vi "Weather Parse Test.vi"() -> ()   [LabVIEW 2020, in "CDM-Config.lvlib"] (continued)
 to 60 NM\\noffshore including San Nicolas and Santa Barbara Islands.\\n\\n* WHEN...From 9 PM this evening to 2 PM PST Thursday.\\n\\n* IMPACTS...Conditions will be hazardous to small craft.\\n\\n* ADDITIONAL DETAILS...See the Coastal Waters Forecast (CWFLOX)\\nfor more.\",\n                \"instruction\": \"Inexperienced mariners, especially those operating smaller\\nvessels, should avoid navigating in hazardous conditions.\",\n                \"response\": \"Avoid\",\n                \"parameters\": {\n                    \"AWIPSidentifier\": [\n                        \"MWWLOX\"\n                    ],\n                    \"WMOidentifier\": [\n                        \"WHUS76 KLOX 031003\"\n                    ],\n                    \"NWSheadline\": [\n                        \"SMALL CRAFT ADVISORY IN EFFECT FROM 9 PM THIS EVENING TO 2 PM PST THURSDAY\"\n                    ],\n                    \"BLOCKCHANNEL\": [\n                        \"EAS\",\n                        \"NWEM\",\n                        \"CMAS\"\n                    ],\n                    \"VTEC\": [\n                        \"/O.NEW.KLOX.SC.Y.0187.251204T0500Z-251204T2200Z/\"\n                    ],\n                    \"eventEndingTime\": [\n                        \"2025-12-04T14:00:00-08:00\"\n                    ]\n                },\n                \"scope\": \"Public\",\n                \"code\": \"IPAWSv1.0\",\n                \"language\": \"en-US\",\n                \"web\": \"http://www.weather.gov\",\n                \"eventCode\": {\n                    \"SAME\": [\n                        \"NWS\"\n                    ],\n                    \"NationalWeatherService\": [\n                        \"SCY\"\n                    ]\n                }\n            }\n        },\n        {\n            \"id\": \"https://api.weather.gov/alerts/urn:oid:2.49.0.1.840.0.b223a23810f154d96d0d97456b98216ffe2bcb9d.002.1\",\n            \"type\": \"Feature\",\n            \"geometry\": null,\n            \"properties\": {\n                \"@id\": \"https://api.weather.gov/alerts/urn:oid:2.49.0.1.840.0.b223a23810f154d96d0d97456b98216ffe2bcb9d.002.1\",\n                \"@type\": \"wx:Alert\",\n                \"id\": \"urn:oid:2.49.0.1.840.0.b223a23810f154d96d0d97456b98216ffe2bcb9d.002.1\",\n                \"areaDesc\": \"Point Piedras Blancas to Point Sal from 10 to 60 NM\",\n                \"geocode\": {\n                    \"SAME\": [\n                        \"057670\"\n                    ],\n                    \"UGC\": [\n                        \"PZZ670\"\n                    ]\n                },\n                \"affectedZones\": [\n                    \"https://api.weather.gov/zones/forecast/PZZ670\"\n                ],\n                \"references\": [\n                    {\n                        \"@id\": \"https://api.weather.gov/alerts/urn:oid:2.49.0.1.840.0.da9279c8d6a996e741e643e2cbd0d5a9445846be.003.1\",\n                        \"identifier\": \"urn:oid:2.49.0.1.840.0.da9279c8d6a996e741e643e2cbd0d5a9445846be.003.1\",\n                        \"sender\": \"w-nws.webmaster@noaa.gov\",\n                        \"sent\": \"2025-12-02T21:13:00-08:00\"\n                    }\n                ],\n                \"sent\": \"2025-12-03T02:03:00-08:00\",\n                \"effective\": \"2025-12-03T02:03:00-08:00\",\n                \"onset\": \"2025-12-03T02:03:00-08:00\",\n                \"expires\": \"2025-12-03T10:00:00-08:00\",\n                \"ends\": \"2025-12-03T10:00:00-08:00\",\n                \"status\": \"Actual\",\n                \"messageType\": \"Update\",\n                \"category\": \"Met\",\n                \"severity\": \"Minor\",\n                \"certainty\": \"Likely\",\n                \"urgency\": \"Expected\",\n                \"event\": \"Small Craft Advisory\",\n                \"sender\": \"w-nws.webmaster@noaa.gov\",\n                \"senderName\": \"NWS Los Angeles/Oxnard CA\",\n                \"headline\": \"Small Craft Advisory issued December 3 at 2:03AM PST until December 3 at 10:00AM PST by NWS Los Angeles/Oxnard CA\",\n                \"description\": \"* WHAT...Hazardous sea conditions.\\n\\n* WHERE...Point Piedras Blancas to Point Sal from 10 to 60 NM.\\n\\n* WHEN...Until 10 AM PST this morning.\\n\\n* IMPACTS...Conditions will be hazardous to small craft.\\n\\n* ADDITIONAL DETAILS...See the Coastal Waters Forecast (CWFLOX)\\nfor more.\",\n                \"instruction\": \"Inexperienced mariners, especially those operating smaller\\nvessels, should avoid navigating in hazardous conditions.\",\n                \"response\": \"Avoid\",\n                \"parameters\": {\n                    \"AWIPSidentifier\": [\n                        \"MWWLOX\"\n                    ],\n                    \"WMOidentifier\": [\n                        \"WHUS76 KLOX 031003\"\n                    ],\n                    \"NWSheadline\": [\n                        \"SMALL CRAFT ADVISORY REMAINS IN EFFECT UNTIL 10 AM PST THIS MORNING\"\n                    ],\n                    \"BLOCKCHANNEL\": [\n                        \"EAS\",\n                        \"NWEM\",\n                        \"CMAS\"\n                    ],\n                    \"VTEC\": [\n                        \"/O.CON.KLOX.SC.Y.0186.000000T0000Z-251203T1800Z/\"\n                    ],\n                    \"eventEndingTime\": [\n                        \"2025-12-03T10:00:00-08:00\"\n                    ],\n                    \"expiredReferences\": [\n                        \"w-nws.webmaster@noaa.gov,urn:oid:2.49.0.1.840.0.03bf4d8e76a679c68e6d6d1c69bed8b6ac358ac0.001.1,2025-12-02T16:31:00-08:00 w-nws.webmaster@noaa.gov,urn:oid:2.49.0.1.840.0.a0fbc3255ee7827afecade81522465af6da1e5e8.001.1,2025-12-02T08:16:00-08:00 w-nws.webmaster@noaa.gov,urn:oid:2.49.0.1.840.0.8e668e000c4ef90085bd20b8852b2e419ef5ec00.001.1,2025-12-02T02:02:00-08:00\"\n                    ]\n                },\n                \"scope\": \"Public\",\n                \"code\": \"IPAWSv1.0\",\n                \"language\": \"en-US\",\n                \"web\": \"http://www.weather.gov\",\n                \"eventCode\": {\n                    \"SAME\": [\n                        \"NWS\"\n                    ],\n                    \"NationalWeatherService\": [\n                        \"SCY\"\n                    ]\n                }\n            }\n        },\n        {\n            \"id\": \"https://api.weather.gov/alerts/urn:oid:2.49.0.1.840.0.71d851f215deadf32c950ba049a11b63260bba93.001.1\",\n            \"type\": \"Feature\",\n            \"geometry\": null,\n            \"properties\": {\n                \"@id\": \"https://api.weather.gov/alerts/urn:oid:2.49.0.1.840.0.71d851f215deadf32c950ba049a11b63260bba93.001.1\",\n                \"@type\": \"wx:Alert\",\n                \"id\": \"urn:oid:2.49.0.1.840.0.71d851f215deadf32c950ba049a11b63260bba93.001.1\",\n                \"areaDesc\": \"Columbia River Bar\",\n                \"geocode\": {\n                    \"SAME\": [\n                        \"057210\"\n                    ],\n                    \"UGC\": [\n                        \"PZZ210\"\n                    ]\n                },\n                \"affectedZones\": [\n                    \"https://api.weather.gov/zones/forecast/PZZ210\"\n                ],\n                \"references\": [],\n                \"sent\": \"2025-12-03T02:01:00-08:00\",\n                \"effective\": \"2025-12-03T02:01:00-08:00\",\n                \"onset\": \"2025-12-03T13:00:00-08:00\",\n                \"expires\": \"2025-12-03T17:00:00-08:00\",\n                \"ends\": \"2025-12-03T17:00:00-08:00\",\n                \"status\": \"Actual\",\n                \"messageType\": \"Alert\",\n                \"category\": \"Met\",\n                \"severity\": \"Minor\",\n                \"certainty\": \"Likely\",\n                \"urgency\": \"Expected\",\n                \"event\": \"Small Craft Advisory\",\n                \"sender\": \"w-nws.webmaster@noaa.gov\",\n                \"senderName\": \"NWS Portland OR\",\n                \"headline\": \"Small Craft Advisory issued December 3 at 2:01AM PST until December 3 at 5:00PM PST by NWS Portland OR\",\n                \"description\": \"* WHAT...Rough bar conditions expected during a very strong ebb\\ncurrent of 7.14 kt at 301 PM Wednesday. Seas 10 ft.\\n\\n* WHERE...In the Main Channel of the Columbia River Bar.\\n\\n* WHEN...From 1 PM to 5 PM PST this afternoon.\\n\\n* IMPACTS...Conditions will be hazardous to small craft,\\nespecially when operating near to, or attempting to cross, the\\nColumbia River Bar.\",\n                \"instruction\": \"A Small Craft Advisory means that wave conditions are expected to\\nbe hazardous to small craft in the vicinity of the Columbia River\\nBar. Mariners are advised to obtain the latest bar conditions\\nfrom the United States Coast Guard before attempting to cross the\\nbar.\",\n                \"response\": \"Avoid\",\n                \"parameters\": {\n                    \"AWIPSidentifier\": [\n                        \"MWWPQR\"\n                    ],\n                    \"WMOidentifier\": [\n                        \"WHUS76 KPQR 031001\"\n                    ],\n                    \"NWSheadline\": [\n                        \"SMALL CRAFT ADVISORY IN EFFECT FROM 1 PM TO 5 PM PST THIS AFTERNOON\"\n                    ],\n                    \"BLOCKCHANNEL\": [\n                        \"EAS\",\n                        \"NWEM\",\n                        \"CMAS\"\n                    ],\n                    \"VTEC\": [\n                        \"/O.NEW.KPQR.SC.Y.0142.251203T2100Z-251204T0100Z/\"\n                    ],\n                    \"eventEndingTime\": [\n                        \"2025-12-03T17:00:00-08:00\"\n                    ]\n                },\n                \"scope\": \"Public\",\n                \"code\": \"IPAWSv1.0\",\n                \"language\": \"en-US\",\n                \"web\": \"http://www.weather.gov\",\n                \"eventCode\": {\n                    \"SAME\": [\n                        \"NWS\"\n                    ],\n                    \"NationalWeatherService\": [\n                        \"SCY\"\n                    ]\n                }\n            }\n        },\n        {\n            \"id\": \"https://api.weather.gov/alerts/urn:oid:2.49.0.1.840.0.b40606fb01e4d94a8ca9e9a27f2c4722d3eb8aec.002.1\",\n            \"type\": \"Feature\",\n            \"geometry\": null,\n            \"properties\": {\n                \"@id\": \"https://api.weather.gov/alerts/urn:oid:2.49.0.1.840.0.b40606fb01e4d94a8ca9e9a27f2c4722d3eb8aec.002.1\",\n                \"@type\": \"wx:Alert\",\n                \"id\": \"urn:oid:2.49.0.1.840.0.b40606fb01e4d94a8ca9e9a27f2c4722d3eb8aec.002.1\",\n                \"areaDesc\": \"Tillamook County Coast; Central Coast of Oregon\",\n                \"geocode\": {\n                    \"SAME\": [\n                        \"041057\",\n                        \"041041\",\n                        \"041039\"\n                    ],\n                    \"UGC\": [\n                        \"ORZ102\",\n                        \"ORZ103\"\n                    ]\n                },\n                \"affectedZones\": [\n                    \"https://api.weather.gov/zones/forecast/ORZ102\",\n                    \"https://api.weather.gov/zones/forecast/ORZ103\"\n                ],\n                \"references\": [\n                    {\n                        \"@id\": \"https://api.weather.gov/alerts/urn:oid:2.49.0.1.840.0.b0d8924765acde472ad27290e55ee6e4f32b14ec.002.1\",\n                        \"identifier\": \"urn:oid:2.49.0.1.840.0.b0d8924765acde472ad27290e55ee6e4f32b14ec.002.1\",\n                        \"sender\": \"w-nws.webmaster@noaa.gov\",\n                        \"sent\": \"2025-12-02T15:12:00-08:00\"\n                    }\n                ],\n                \"sent\": \"2025-12-03T02:01:00-08:00\",\n                \"effective\": \"2025-12-03T02:01:00-08:00\",\n                \"onset\": \"2025-12-03T02:01:00-08:00\",\n                \"expires\": \"2025-12-03T22:00:00-08:00\",\n                \"ends\": \"2025-12-03T22:00:00-08:00\",\n                \"status\": \"Actual\",\n                \"messageType\": \"Update\",\n                \"category\": \"Met\",\n                \"severity\": \"Moderate\",\n                \"certainty\": \"Likely\",\n                \"urgency\": \"Expected\",\n                \"event\": \"Beach Hazards Statement\",\n                \"sender\": \"w-nws.webmaster@noaa.gov\",\n                \"senderName\": \"NWS Portland OR\",\n                \"headline\": \"Beach Hazards Statement issued December 3 at 2:01AM PST until December 3 at 10:00PM PST by NWS Portland OR\",\n                \"description\": \"* WHAT...Sneaker waves possible.\\n\\n* WHERE...Tillamook County Coast and Central Coast of Oregon.\\n\\n* WHEN...Through this evening.\\n\\n* IMPACTS...Waves can run up significantly farther on a beach\\nthan normal, including over rocks and jetties. Sneaker waves\\ncan suddenly knock beachgoers off if their feet and quickly\\npull them into the frigid ocean which may lead to serious\\ninjury or drowning.\\n\\n* ADDITIONAL DETAILS...A Beach Hazards Statement is issued when\\nsneaker waves create potentially life-threatening conditions\\nin the surf zone. Caution should be used when in or near the\\nwater. Always keep an eye on the waves, and be especially\\nwatchful of children. Those participating in razor clam digs\\nshould additionally exercise caution.\",\n                \"instruction\": \"Remain out of the water to avoid hazardous swimming conditions.\",\n                \"response\": \"Avoid\",\n                \"parameters\": {\n                    \"AWIPSidentifier\": [\n                        \"CFWPQR\"\n                    ],\n                    \"WMOidentifier\": [\n                        \"WHUS46 KPQR 031001\"\n                    ],\n                    \"NWSheadline\": [\n                        \"BEACH HAZARDS STATEMENT REMAINS IN EFFECT THROUGH THIS EVENING\"\n                    ],\n                    \"BLOCKCHANNEL\": [\n                        \"EAS\",\n                        \"NWEM\",\n                        \"CMAS\"\n                    ],\n                    \"VTEC\": [\n                        \"/O.CON.KPQR.BH.S.0016.000000T0000Z-251204T0600Z/\"\n                    ],\n                    \"eventEndingTime\": [\n                        \"2025-12-03T22:00:00-08:00\"\n                    ],\n                    \"expiredReferences\": [\n                        \"w-nws.webmaster@noaa.gov,urn:oid:2.49.0.1.840.0.4a86d466bdedede9df987ed309d495de11850650.001.1,2025-12-01T14:28:00-08:00 w-nws.webmaster@noaa.gov,urn:oid:2.49.0.1.840.0.7f5d42e9aa955b7ce231997bb6cbc5205d11387b.001.1,2025-11-30T13:55:00-08:00 w-nws.webmaster@noaa.gov,urn:oid:2.49.0.1.840.0.f9f5603af29c238f0de04ac7e2a9349708c05a53.001.1,2025-11-29T13:40:00-08:00 w-nws.webmaster@noaa.gov,urn:oid:2.49.0.1.840.0.5d50b6fb5ef96869ff9b56cca9e1ba6ccd50c4dd.001.1,2025-11-28T14:00:00-08:00\"\n                    ]\n                },\n                \"scope\": \"Public\",\n                \"code\": \"IPAWSv1.0\",\n                \"language\": \"en-US\",\n                \"web\": \"http://www.weather.gov\",\n                \"eventCode\": {\n                    \"SAME\": [\n                        \"NWS\"\n                    ],\n                    \"NationalWeatherService\": [\n                        \"BHS\"\n                    ]\n                }\n            }\n        },\n        {\n            \"id\": \"https://api.weather.gov/alerts/urn:oid:2.49.0.1.840.0.b40606fb01e4d94a8ca9e9a27f2c4722d3eb8aec.001.1\",\n            \"type\": \"Feature\",\n            \"geometry\": null,\n            \"properties\": {\n                \"@id\": \"https://api.weather.gov/alerts/urn:oid:2.49.0.1.840.0.b40606fb01e4d94a8ca9e9a27f2c4722d3eb8aec.001.1\",\n                \"@type\": \"wx:Alert\",\n                \"id\": \"urn:oid:2.49.0.1.840.0.b40606fb01e4d94a8ca9e9a27f2c4722d3eb8aec.001.1\",\n                \"areaDesc\": \"Clatsop County Coast; South Washington Coast\",\n                \"geocode\": {\n                    \"SAME\": [\n                        \"041007\",\n                        \"053049\"\n                    ],\n                    \"UGC\": [\n                        \"ORZ101\",\n                        \"WAZ201\"\n                    ]\n                },\n                \"affectedZones\": [\n                    \"https://api.weather.gov/zones/forecast/ORZ101\",\n                    \"https://api.weather.gov/zones/forecast/WAZ201\"\n                ],\n                \"references\": [\n                    {\n                        \"@id\": \"https://api.weather.gov/alerts/urn:oid:2.49.0.1.840.0.b0d8924765acde472ad27290e55ee6e4f32b14ec.001.1\",\n                        \"identifier\": \"urn:oid:2.49.0.1.840.0.b0d8924765acde472ad27290e55ee6e4f32b14ec.001.1\",\n                        \"sender\": \"w-nws.webmaster@noaa.gov\",\n                        \"sent\": \"2025-12-02T15:12:00-08:00\"\n                    }\n                ],\n                \"sent\": \"2025-12-03T02:01:00-08:00\",\n                \"effective\": \"2025-12-03T02:01:00-08:00\",\n                \"onset\": \"2025-12-04T09:00:00-08:00\",\n                \"expires\": \"2025-12-03T22:00:00-08:00\",\n                \"ends\": \"2025-12-04T14:00:00-08:00\",\n                \"status\": \"Actual\",\n                \"messageType\": \"Update\",\n                \"category\": \"Met\",\n                \"severity\": \"Minor\",\n                \"certainty\": \"Likely\",\n                \"urgency\": \"Expected\",\n                \"event\": \"Coastal Flood Advisory\",\n                \"sender\": \"w-nws.webmaster@noaa.gov\",\n                \"senderName\": \"NWS Portland OR\",\n                \"headline\": \"Coastal Flood Advisory issued December 3 at 2:01AM PST until December 4 at 2:00PM PST by NWS Portland OR\",\n                \"description\": \"* WHAT...For the Beach Hazards Statement, Sneaker waves\\npossible. For the Coastal Flood Advisory, tidal overflow\\nflooding expected.\\n\\n* WHERE...In Oregon, Clatsop County Coast. In Washington, South\\nWashington Coast.\\n\\n* WHEN...For the Beach Hazards Statement, through this evening.\\nFor the Coastal Flood Advisory, from 9 AM to 2 PM PST Thursday.\\n\\n* IMPACTS...Waves can run up significantly farther on a beach\\nthan normal, including over rocks and jetties. Sneaker waves\\ncan suddenly knock beachgoers off if their feet and quickly\\npull them into the frigid ocean which may lead to serious\\ninjury or drowning.\\n\\nFor the Coastal Flood Advisory, minor flooding is possible in\\nlow lying areas near bays, sloughs, and the lower reaches of\\nthe coastal rivers. This is due to total tide of up to 11.1\\nfeet at Toke Point resulting in tide up to one foot above\\nground level during high tide, total tide of up to 10.6 feet\\nat Tongue Point resulting in tide up to one foot above ground\\nlevel.\\n\\n* ADDITIONAL DETAILS...A Beach Hazards Statement is issued when\\nsneaker waves create potentially life-threatening conditions\\nin the surf zone. Caution should be used when in or near the\\nwater. Always keep an eye on the waves, and be especially\\nwatchful of children. Those participating in razor clam digs\\nshould additionally exercise caution.\",\n                \"instruction\": \"A Coastal Flood Advisory means that tidal overflow flooding is\\nexpected. Coastal residents in the warned area should be alert\\nfor rising water, and take appropriate action to protect life and\\nproperty.\\n\\nRemain out of the water to avoid hazardous swimming conditions.\",\n                \"response\": \"Monitor\",\n                \"parameters\": {\n                    \"AWIPSidentifier\": [\n                        \"CFWPQR\"\n                    ],\n                    \"WMOidentifier\": [\n                        \"WHUS46 KPQR 031001\"\n                    ],\n                    \"NWSheadline\": [\n                        \"BEACH HAZARDS STATEMENT REMAINS IN EFFECT THROUGH THIS EVENING... ...COASTAL FLOOD ADVISORY REMAINS IN EFFECT FROM 9 AM TO 2 PM PST THURSDAY\"\n                    ],\n                    \"BLOCKCHANNEL\": [\n                        \"EAS\",\n                        \"NWEM\",\n                        \"CMAS\"\n                    ],\n                    \"VTEC\": [\n                        \"/O.CON.KPQR.CF.Y.0005.251204T1700Z-251204T2200Z/\"\n                    ],\n                    \"eventEndingTime\": [\n                        \"2025-12-04T14:00:00-08:00\"\n                    ]\n                },\n                \"scope\": \"Public\",\n                \"code\": \"IPAWSv1.0\",\n                \"language\": \"en-US\",\n                \"web\": \"http://www.weather.gov\",\n                \"eventCode\": {\n                    \"SAME\": [\n                        \"NWS\"\n                    ],\n                    \"NationalWeatherService\": [\n                        \"CFY\"\n                    ]\n                }\n            }\n        },\n        {\n            \"id\": \"https://api.weather.gov/alerts/urn:oid:2.49.0.1.840.0.b40606fb01e4d94a8ca9e9a27f2c4722d3eb8aec.001.2\",\n            \"type\": \"Feature\",\n            \"geometry\": null,\n            \"properties\": {\n                \"@id\": \"https://api.weather.gov/alerts/urn:oid:2.49.0.1.840.0.b40606fb01e4d94a8ca9e9a27f2c4722d3eb8aec.001.2\",\n                \"@type\": \"wx:Alert\",\n                \"id\": \"urn:oid:2.49.0.1.840.0.b40606fb01e4d94a8ca9e9a27f2c4722d3eb8aec.001.2\",\n                \"areaDesc\": \"Clatsop County Coast; South Washington Coast\",\n                \"geocode\": {\n                    \"SAME\": [\n                        \"041007\",\n                        \"053049\"\n                    ],\n                    \"UGC\": [\n                        \"ORZ101\",\n                        \"WAZ201\"\n                    ]\n                },\n                \"affectedZones\": [\n                    \"https://api.weather.gov/zones/forecast/ORZ101\",\n                    \"https://api.weather.gov/zones/forecast/WAZ201\"\n                ],\n                \"references\": [\n                    {\n                        \"@id\": \"https://api.weather.gov/alerts/urn:oid:2.49.0.1.840.0.b0d8924765acde472ad27290e55ee6e4f32b14ec.001.2\",\n                        \"identifier\": \"urn:oid:2.49.0.1.840.0.b0d8924765acde472ad27290e55ee6e4f32b14ec.001.2\",\n                        \"sender\": \"w-nws.webmaster@noaa.gov\",\n                        \"sent\": \"2025-12-02T15:12:00-08:00\"\n                    }\n                ],\n                \"sent\": \"2025-12-03T02:01:00-08:00\",\n                \"effective\": \"2025-12-03T02:01:00-08:00\",\n                \"onset\": \"2025-12-03T02:01:00-08:00\",\n                \"expires\": \"2025-12-03T22:00:00-08:00\",\n                \"ends\": \"2025-12-03T22:00:00-08:00\",\n                \"status\": \"Actual\",\n                \"messageType\": \"Update\",\n                \"category\": \"Met\",\n                \"severity\": \"Moderate\",\n                \"certainty\": \"Likely\",\n                \"urgency\": \"Expected\",\n                \"event\": \"Beach Hazards Statement\",\n                \"sender\": \"w-nws.webmaster@noaa.gov\",\n                \"senderName\": \"NWS Portland OR\",\n                \"headline\": \"Beach Hazards Statement issued December 3 at 2:01AM PST until December 3 at 10:00PM PST by NWS Portland OR\",\n                \"description\": \"* WHAT...For the Beach Hazards Statement, Sneaker waves\\npossible. For the Coastal Flood Advisory, tidal overflow\\nflooding expected.\\n\\n* WHERE...In Oregon, Clatsop County Coast. In Washington, South\\nWashington Coast.\\n\\n* WHEN...For the Beach Hazards Statement, through this evening.\\nFor the Coastal Flood Advisory, from 9 AM to 2 PM PST Thursday.\\n\\n* IMPACTS...Waves can run up significantly farther on a beach\\nthan normal, including over rocks and jetties. Sneaker waves\\ncan suddenly knock beachgoers off if their feet and quickly\\npull them into the frigid ocean which may lead to serious\\ninjury or drowning.\\n\\nFor the Coastal Flood Advisory, minor flooding is possible in\\nlow lying areas near bays, sloughs, and the lower reaches of\\nthe coastal rivers. This is due to total tide of up to 11.1\\nfeet at Toke Point resulting in tide up to one foot above\\nground level during high tide, total tide of up to 10.6 feet\\nat Tongue Point resulting in tide up to one foot above ground\\nlevel.\\n\\n* ADDITIONAL DETAILS...A Beach Hazards Statement is issued when\\nsneaker waves create potentially life-threatening conditions\\nin the surf zone. Caution should be used when in or near the\\nwater. Always keep an eye on the waves, and be especially\\nwatchful of children. Those participating in razor clam digs\\nshould additionally exercise caution.\",\n                \"instruction\": \"A Coastal Flood Advisory means that tidal overflow flooding is\\nexpected. Coastal residents in the warned area should be alert\\nfor rising water, and take appropriate action to protect life and\\nproperty.\\n\\nRemain out of the water to avoid hazardous swimming conditions.\",\n                \"response\": \"Avoid\",\n                \"parameters\": {\n                    \"AWIPSidentifier\": [\n                        \"CFWPQR\"\n                    ],\n                    \"WMOidentifier\": [\n                        \"WHUS46 KPQR 031001\"\n                    ],\n                    \"NWSheadline\": [\n                        \"BEACH HAZARDS STATEMENT REMAINS IN EFFECT THROUGH THIS EVENING... ...COASTAL FLOOD ADVISORY REMAINS IN EFFECT FROM 9 AM TO 2 PM PST THURSDAY\"\n                    ],\n                    \"BLOCKCHANNEL\": [\n                        \"EAS\",\n                        \"NWEM\",\n                        \"CMAS\"\n                    ],\n                    \"VTEC\": [\n                        \"/O.CON.KPQR.BH.S.0016.000000T0000Z-251204T0600Z/\"\n                    ],\n                    \"eventEndingTime\": [\n                        \"2025-12-03T22:00:00-08:00\"\n                    ],\n                    \"expiredReferences\": [\n                        \"w-nws.webmaster@noaa.gov,urn:oid:2.49.0.1.840.0.4a86d466bdedede9df987ed309d495de11850650.001.1,2025-12-01T14:28:00-08:00 w-nws.webmaster@noaa.gov,urn:oid:2.49.0.1.840.0.7f5d42e9aa955b7ce231997bb6cbc5205d11387b.001.1,2025-11-30T13:55:00-08:00 w-nws.webmaster@noaa.gov,urn:oid:2.49.0.1.840.0.f9f5603af29c238f0de04ac7e2a9349708c05a53.001.1,2025-11-29T13:40:00-08:00 w-nws.webmaster@noaa.gov,urn:oid:2.49.0.1.840.0.5d50b6fb5ef96869ff9b56cca9e1ba6ccd50c4dd.001.1,2025-11-28T14:00:00-08:00\"\n                    ]\n                },\n                \"scope\": \"Public\",\n                \"code\": \"IPAWSv1.0\",\n                \"language\": \"en-US\",\n                \"web\": \"http://www.weather.gov\",\n                \"eventCode\": {\n                    \"SAME\": [\n                        \"NWS\"\n                    ],\n                    \"NationalWeatherService\": [\n                        \"BHS\"\n                    ]\n                }\n            }\n        },\n        {\n            \"id\": \"https://api.weather.gov/alerts/urn:oid:2.49.0.1.840.0.59f39e0a7f6acf285dcd268db360e347a0a8a808.001.2\",\n            \"type\": \"Feature\",\n            \"geometry\": null,\n            \"properties\": {\n                \"@id\": \"https://api.weather.gov/alerts/urn:oid:2.49.0.1.840.0.59f39e0a7f6acf285dcd268db360e347a0a8a808.001.2\",\n                \"@type\": \"wx:Alert\",\n                \"id\": \"urn:oid:2.49.0.1.840.0.59f39e0a7f6acf285dcd268db360e347a0a8a808.001.2\",\n                \"areaDesc\": \"Ventura County Beaches\",\n                \"geocode\": {\n                    \"SAME\": [\n                        \"006111\"\n                    ],\n                    \"UGC\": [\n                        \"CAZ354\"\n                    ]\n                },\n                \"affectedZones\": [\n                    \"https://api.weather.gov/zones/forecast/CAZ354\"\n                ],\n                \"references\": [\n                    {\n                        \"@id\": \"https://api.weather.gov/alerts/urn:oid:2.49.0.1.840.0.93417926f6a4e3b4090235b97e1fee71b07b4e44.001.2\",\n                        \"identifier\": \"urn:oid:2.49.0.1.840.0.93417926f6a4e3b4090235b97e1fee71b07b4e44.001.2\",\n                        \"sender\": \"w-nws.webmaster@noaa.gov\",\n                        \"sent\": \"2025-12-02T13:27:00-08:00\"\n                    }\n                ],\n                \"sent\": \"2025-12-03T02:00:00-08:00\",\n                \"effective\": \"2025-12-03T02:00:00-08:00\",\n                \"onset\": \"2025-12-03T03:00:00-08:00\",\n                \"expires\": \"2025-12-03T10:00:00-08:00\",\n                \"ends\": \"2025-12-03T10:00:00-08:00\",\n                \"status\": \"Actual\",\n                \"messageType\": \"Update\",\n                \"category\": \"Met\",\n                \"severity\": \"Minor\",\n                \"certainty\": \"Likely\",\n                \"urgency\": \"Expected\",\n                \"event\": \"Coastal Flood Advisory\",\n                \"sender\": \"w-nws.webmaster@noaa.gov\",\n                \"senderName\": \"NWS Los Angeles/Oxnard CA\",\n                \"headline\": \"Coastal Flood Advisory issued December 3 at 2:00AM PST until December 3 at 10:00AM PST by NWS Los Angeles/Oxnard CA\",\n                \"description\": \"* WHAT...For the High Surf Advisory, large breaking waves of 4 to\\n7 feet. Dangerous rip currents expected. For the Coastal Flood\\nAdvisory, minor coastal flooding is possible during high tide.\\n\\n* WHERE...Ventura County Beaches.\\n\\n* WHEN...For the High Surf Advisory, until noon PST Thursday.\\nFor the Coastal Flood Advisory, until 10 AM PST this morning.\\n\\n* IMPACTS...Flooding of sea water is likely, around the time of\\nhigh tide, over vulnerable low-lying coastal areas such as\\nparking lots, beaches, and walkways. Significant damage to roads\\nor structures is NOT expected. There is an increased risk for\\nocean drowning. Rip currents can pull swimmers and surfers out\\nto sea. Large breaking waves can cause injury, wash people off\\nbeaches and rocks, and capsize small boats near shore.\",\n                \"instruction\": \"Take the necessary actions to protect flood-prone property. Do\\nNOT drive around barricades or through water of unknown depth.\\n\\nRemain out of the water due to dangerous surf conditions, or stay\\nnear occupied lifeguard towers. Rock jetties can be deadly in\\nsuch conditions, stay off the rocks.\",\n                \"response\": \"Monitor\",\n                \"parameters\": {\n                    \"AWIPSidentifier\": [\n                        \"CFWLOX\"\n                    ],\n                    \"WMOidentifier\": [\n                        \"WHUS46 KLOX 031000\"\n                    ],\n                    \"NWSheadline\": [\n                        \"HIGH SURF ADVISORY REMAINS IN EFFECT UNTIL NOON PST THURSDAY... ...COASTAL FLOOD ADVISORY REMAINS IN EFFECT UNTIL 10 AM PST THIS MORNING\"\n                    ],\n                    \"BLOCKCHANNEL\": [\n                        \"EAS\",\n                        \"NWEM\",\n                        \"CMAS\"\n                    ],\n                    \"VTEC\": [\n                        \"/O.CON.KLOX.CF.Y.0004.251203T1100Z-251203T1800Z/\"\n                    ],\n                    \"eventEndingTime\": [\n                        \"2025-12-03T10:00:00-08:00\"\n                    ],\n                    \"expiredReferences\": [\n                        \"w-nws.webmaster@noaa.gov,urn:oid:2.49.0.1.840.0.2ef03bba301f3aa5d410947a3c0b158da4ab8a14.001.2,2025-12-02T01:44:00-08:00 w-nws.webmaster@noaa.gov,urn:oid:2.49.0.1.840.0.ca1df4acb1d2f6b371b32e7cbfbf7966eb5b8a28.001.2,2025-12-01T19:11:00-08:00 w-nws.webmaster@noaa.gov,urn:oid:2.49.0.1.840.0.9f5f82a93112b0fbb919461d7f3c09a028cde467.001.1,2025-12-01T12:55:00-08:00\"\n                    ]\n                },\n                \"scope\": \"Public\",\n                \"code\": \"IPAWSv1.0\",\n                \"language\": \"en-US\",\n                \"web\": \"http://www.weather.gov\",\n                \"eventCode\": {\n                    \"SAME\": [\n                        \"NWS\"\n                    ],\n                    \"NationalWeatherService\": [\n                        \"CFY\"\n                    ]\n                }\n            }\n        },\n        {\n            \"id\": \"https://api.weather.gov/alerts/urn:oid:2.49.0.1.840.0.59f39e0a7f6acf285dcd268db360e347a0a8a808.003.1\",\n            \"type\": \"Feature\",\n            \"geometry\": null,\n            \"properties\": {\n                \"@id\": \"https://api.weather.gov/alerts/urn:oid:2.49.0.1.840.0.59f39e0a7f6acf285dcd268db360e347a0a8a808.003.1\",\n                \"@type\": \"wx:Alert\",\n                \"id\": \"urn:oid:2.49.0.1.840.0.59f39e0a7f6acf285dcd268db360e347a0a8a808.003.1\",\n                \"areaDesc\": \"Santa Barbara County Southwestern Coast; Santa Barbara County Southeastern Coast; Malibu Coast; Los Angeles County Beaches\",\n                \"geocode\": {\n                    \"SAME\": [\n                        \"006083\",\n                        \"006037\"\n                    ],\n                    \"UGC\": [\n                        \"CAZ349\",\n                        \"CAZ350\",\n                        \"CAZ362\",\n                        \"CAZ366\"\n                    ]\n                },\n                \"affectedZones\": [\n                    \"https://api.weather.gov/zones/forecast/CAZ349\",\n                    \"https://api.weather.gov/zones/forecast/CAZ350\",\n                    \"https://api.weather.gov/zones/forecast/CAZ362\",\n                    \"https://api.weather.gov/zones/forecast/CAZ366\"\n                ],\n                \"references\": [\n                    {\n                        \"@id\": \"https://api.weather.gov/alerts/urn:oid:2.49.0.1.840.0.93417926f6a4e3b4090235b97e1fee71b07b4e44.003.1\",\n                        \"identifier\": \"urn:oid:2.49.0.1.840.0.93417926f6a4e3b4090235b97e1fee71b07b4e44.003.1\",\n                        \"sender\": \"w-nws.webmaster@noaa.gov\",\n                        \"sent\": \"2025-12-02T13:27:00-08:00\"\n                    }\n                ],\n                \"sent\": \"2025-12-03T02:00:00-08:00\",\n                \"effective\": \"2025-12-03T02:00:00-08:00\",\n                \"onset\": \"2025-12-03T02:00:00-08:00\",\n                \"expires\": \"2025-12-03T10:00:00-08:00\",\n                \"ends\": \"2025-12-06T11:00:00-08:00\",\n                \"status\": \"Actual\",\n                \"messageType\": \"Update\",\n                \"category\": \"Met\",\n                \"severity\": \"Moderate\",\n                \"certainty\": \"Likely\",\n                \"urgency\": \"Expected\",\n                \"event\": \"Beach Hazards Statement\",\n                \"sender\": \"w-nws.webmaster@noaa.gov\",\n                \"senderName\": \"NWS Los Angeles/Oxnard CA\",\n                \"headline\": \"Beach Hazards Statement issued December 3 at 2:00AM PST until December 6 at 11:00AM PST by NWS Los Angeles/Oxnard CA\",\n                \"description\": \"* WHAT...Dangerous rip currents and breaking waves due to\\nelevated surf expected. Minor tidal overflows are possible\\nfrom 4 AM to 12 PM each day through Saturday morning.\\n\\n* WHERE...Santa Barbara County Southwestern Coast, Santa Barbara\\nCounty Southeastern Coast, Malibu Coast and Los Angeles County\\nBeaches.\\n\\n* WHEN...Through Saturday morning.\\n\\n* IMPACTS...There is an increased risk of ocean drowning. Rip\\ncurrents can pull swimmers and surfers out to sea. Waves can\\nwash people off beaches and rocks, and capsize small boats\\nnearshore.\\n\\n* ADDITIONAL DETAILS... Elevated surf will be highest through\\nThursday.\",\n                \"instruction\": \"Remain out of the water due to hazardous swimming conditions, or\\nstay near occupied lifeguard towers. Rock jetties can be deadly\\nin such conditions, stay off the rocks.\",\n                \"response\": \"Avoid\",\n                \"parameters\": {\n                    \"AWIPSidentifier\": [\n                        \"CFWLOX\"\n                    ],\n                    \"WMOidentifier\": [\n                        \"WHUS46 KLOX 031000\"\n                    ],\n                    \"NWSheadline\": [\n                        \"BEACH HAZARDS STATEMENT REMAINS IN EFFECT THROUGH SATURDAY MORNING\"\n                    ],\n                    \"BLOCKCHANNEL\": [\n                        \"EAS\",\n                        \"NWEM\",\n                        \"CMAS\"\n                    ],\n                    \"VTEC\": [\n                        \"/O.CON.KLOX.BH.S.0018.000000T0000Z-251206T1900Z/\"\n                    ],\n                    \"eventEndingTime\": [\n                        \"2025-12-06T11:00:00-08:00\"\n                    ],\n                    \"expiredReferences\": [\n                        \"w-nws.webmaster@noaa.gov,urn:oid:2.49.0.1.840.0.2ef03bba301f3aa5d410947a3c0b158da4ab8a14.003.1,2025-12-02T01:44:00-08:00 w-nws.webmaster@noaa.gov,urn:oid:2.49.0.1.840.0.ca1df4acb1d2f6b371b32e7cbfbf7966eb5b8a28.003.1,2025-12-01T19:11:00-08:00 w-nws.webmaster@noaa.gov,urn:oid:2.49.0.1.840.0.9f5f82a93112b0fbb919461d7f3c09a028cde467.003.1,2025-12-01T12:55:00-08:00\"\n                    ]\n                },\n                \"scope\": \"Public\",\n                \"code\": \"IPAWSv1.0\",\n                \"language\": \"en-US\",\n                \"web\": \"http://www.weather.gov\",\n                \"eventCode\": {\n                    \"SAME\": [\n                        \"NWS\"\n                    ],\n                    \"NationalWeatherService\": [\n                        \"BHS\"\n                    ]\n                }\n            }\n        },\n        {\n            \"id\": \"https://api.weather.gov/alerts/urn:oid:2.49.0.1.840.0.59f39e0a7f6acf285dcd268db360e347a0a8a808.002.1\",\n            \"type\": \"Feature\",\n            \"geometry\": null,\n            \"properties\": {\n                \"@id\": \"https://api.weather.gov/alerts/urn:oid:2.49.0.1.840.0.59f39e0a7f6acf285dcd268db360e347a0a8a808.002.1\",\n                \"@type\": \"wx:Alert\",\n                \"id\": \"urn:oid:2.49.0.1.840.0.59f39e0a7f6acf285dcd268db360e347a0a8a808.002.1\",\n                \"areaDesc\": \"San Luis Obispo County Beaches; Santa Barbara County Central Coast Beaches\",\n                \"geocode\": {\n                    \"SAME\": [\n                        \"006079\",\n                        \"006083\"\n                    ],\n                    \"UGC\": [\n                        \"CAZ340\",\n                        \"CAZ346\"\n                    ]\n                },\n                \"affectedZones\": [\n                    \"https://api.weather.gov/zones/forecast/CAZ340\",\n                    \"https://api.weather.gov/zones/forecast/CAZ346\"\n                ],\n                \"references\": [\n                    {\n                        \"@id\": \"https://api.weather.gov/alerts/urn:oid:2.49.0.1.840.0.93417926f6a4e3b4090235b97e1fee71b07b4e44.002.1\",\n                        \"identifier\": \"urn:oid:2.49.0.1.840.0.93417926f6a4e3b4090235b97e1fee71b07b4e44.002.1\",\n                        \"sender\": \"w-nws.webmaster@noaa.gov\",\n                        \"sent\": \"2025-12-02T13:27:00-08:00\"\n                    }\n                ],\n                \"sent\": \"2025-12-03T02:00:00-08:00\",\n                \"effective\": \"2025-12-03T02:00:00-08:00\",\n                \"onset\": \"2025-12-03T02:00:00-08:00\",\n                \"expires\": \"2025-12-03T10:00:00-08:00\",\n                \"ends\": \"2025-12-04T03:00:00-08:00\",\n                \"status\": \"Actual\",\n                \"messageType\": \"Update\",\n                \"category\": \"Met\",\n                \"severity\": \"Minor\",\n                \"certainty\": \"Likely\",\n                \"urgency\": \"Expected\",\n                \"event\": \"High Surf Advisory\",\n                \"sender\": \"w-nws.webmaster@noaa.gov\",\n                \"senderName\": \"NWS Los Angeles/Oxnard CA\",\n                \"headline\": \"High Surf Advisory issued December 3 at 2:00AM PST until December 4 at 3:00AM PST by NWS Los Angeles/Oxnard CA\",\n                \"description\": \"* WHAT...Large breaking waves 8 to 12 feet with dangerous rip\\ncurrents. Minor tidal overflows are possible from 4 AM to 11\\nAM Tuesday and Wednesday due to unusually high tides.\\n\\n* WHERE...San Luis Obispo County Beaches and Santa Barbara\\nCounty Central Coast Beaches.\\n\\n* WHEN...Until 3 AM PST Thursday.\\n\\n* IMPACTS...There is an increased risk for ocean drowning. Rip\\ncurrents can pull swimmers and surfers out to sea. Large\\nbreaking waves can cause injury, wash people off beaches and\\nrocks, and capsize small boats near shore.\",\n                \"instruction\": \"Remain out of the water due to dangerous surf conditions, or stay\\nnear occupied lifeguard towers. Rock jetties can be deadly in\\nsuch conditions, stay off the rocks.\",\n                \"response\": \"Avoid\",\n                \"parameters\": {\n                    \"AWIPSidentifier\": [\n                        \"CFWLOX\"\n                    ],\n                    \"WMOidentifier\": [\n                        \"WHUS46 KLOX 031000\"\n                    ],\n                    \"NWSheadline\": [\n                        \"HIGH SURF ADVISORY REMAINS IN EFFECT UNTIL 3 AM PST THURSDAY\"\n                    ],\n                    \"BLOCKCHANNEL\": [\n                        \"EAS\",\n                        \"NWEM\",\n                        \"CMAS\"\n                    ],\n                    \"VTEC\": [\n                        \"/O.CON.KLOX.SU.Y.0028.000000T0000Z-251204T1100Z/\"\n                    ],\n                    \"eventEndingTime\": [\n                        \"2025-12-04T03:00:00-08:00\"\n                    ],\n                    \"expiredReferences\": [\n                        \"w-nws.webmaster@noaa.gov,urn:oid:2.49.0.1.840.0.2ef03bba301f3aa5d410947a3c0b158da4ab8a14.002.1,2025-12-02T01:44:00-08:00 w-nws.webmaster@noaa.gov,urn:oid:2.49.0.1.840.0.ca1df4acb1d2f6b371b32e7cbfbf7966eb5b8a28.002.1,2025-12-01T19:11:00-08:00 w-nws.webmaster@noaa.gov,urn:oid:2.49.0.1.840.0.9f5f82a93112b0fbb919461d7f3c09a028cde467.002.1,2025-12-01T12:55:00-08:00 w-nws.webmaster@noaa.gov,urn:oid:2.49.0.1.840.0.015922fdf015473aef5e5f47db7c0e51f90d6741.001.1,2025-12-01T07:34:00-08:00 w-nws.webmaster@noaa.gov,urn:oid:2.49.0.1.840.0.d822971e3d114269ffa138599ce2d4a4601851da.001.1,2025-12-01T01:55:00-08:00 w-nws.webmaster@noaa.gov,urn:oid:2.49.0.1.840.0.10a9c2b4750f9405598093ce56483ab9d8199c67.002.1,2025-11-30T21:47:00-08:00 w-nws.webmaster@noaa.gov,urn:oid:2.49.0.1.840.0.10a9c2b4750f9405598093ce56483ab9d8199c67.001.1,2025-11-30T21:47:00-08:00 w-nws.webmaster@noaa.gov,urn:oid:2.49.0.1.840.0.57e5fa524eb4c8f2b85a01695262fcb598f7b61e.001.1,2025-11-30T12:57:00-08:00\"\n                    ]\n                },\n                \"scope\": \"Public\",\n                \"code\": \"IPAWSv1.0\",\n                \"language\": \"en-US\",\n                \"web\": \"http://www.weather.gov\",\n                \"eventCode\": {\n                    \"SAME\": [\n                        \"NWS\"\n                    ],\n                    \"NationalWeatherService\": [\n                        \"SUY\"\n                    ]\n                }\n            }\n        },\n        {\n            \"id\": \"https://api.weather.gov/alerts/urn:oid:2.49.0.1.840.0.59f39e0a7f6acf285dcd268db360e347a0a8a808.001.1\",\n            \"type\": \"Feature\",\n            \"geometry\": null,\n            \"properties\": {\n                \"@id\": \"https://api.weather.gov/alerts/urn:oid:2.49.0.1.840.0.59f39e0a7f6acf285dcd268db360e347a0a8a808.001.1\",\n                \"@type\": \"wx:Alert\",\n                \"id\": \"urn:oid:2.49.0.1.840.0.59f39e0a7f6acf285dcd268db360e347a0a8a808.001.1\",\n                \"areaDesc\": \"Ventura County Beaches\",\n                \"geocode\": {\n                    \"SAME\": [\n                        \"006111\"\n                    ],\n                    \"UGC\": [\n                        \"CAZ354\"\n                    ]\n                },\n                \"affectedZones\": [\n                    \"https://api.weather.gov/zones/forecast/CAZ354\"\n                ],\n                \"references\": [\n                    {\n                        \"@id\": \"https://api.weather.gov/alerts/urn:oid:2.49.0.1.840.0.93417926f6a4e3b4090235b97e1fee71b07b4e44.001.1\",\n                        \"identifier\": \"urn:oid:2.49.0.1.840.0.93417926f6a4e3b4090235b97e1fee71b07b4e44.001.1\",\n                        \"sender\": \"w-nws.webmaster@noaa.gov\",\n                        \"sent\": \"2025-12-02T13:27:00-08:00\"\n                    }\n                ],\n                \"sent\": \"2025-12-03T02:00:00-08:00\",\n                \"effective\": \"2025-12-03T02:00:00-08:00\",\n                \"onset\": \"2025-12-03T02:00:00-08:00\",\n                \"expires\": \"2025-12-03T10:00:00-08:00\",\n                \"ends\": \"2025-12-04T12:00:00-08:00\",\n                \"status\": \"Actual\",\n                \"messageType\": \"Update\",\n                \"category\": \"Met\",\n                \"severity\": \"Minor\",\n                \"certainty\": \"Likely\",\n                \"urgency\": \"Expected\",\n                \"event\": \"High Surf Advisory\",\n                \"sender\": \"w-nws.webmaster@noaa.gov\",\n                \"senderName\": \"NWS Los Angeles/Oxnard CA\",\n                \"headline\": \"High Surf Advisory issued December 3 at 2:00AM PST until December 4 at 12:00PM PST by NWS Los Angeles/Oxnard CA\",\n                \"description\": \"* WHAT...For the High Surf Advisory, large breaking waves of 4 to\\n7 feet. Dangerous rip currents expected. For the Coastal Flood\\nAdvisory, minor coastal flooding is possible during high tide.\\n\\n* WHERE...Ventura County Beaches.\\n\\n* WHEN...For the High Surf Advisory, until noon PST Thursday.\\nFor the Coastal Flood Advisory, until 10 AM PST this morning.\\n\\n* IMPACTS...Flooding of sea water is likely, around the time of\\nhigh tide, over vulnerable low-lying coastal areas such as\\nparking lots, beaches, and walkways. Significant damage to roads\\nor structures is NOT expected. There is an increased risk for\\nocean drowning. Rip currents can pull swimmers and surfers out\\nto sea. Large breaking waves can cause injury, wash people off\\nbeaches and rocks, and capsize small boats near shore.\",\n                \"instruction\": \"Take the necessary actions to protect flood-prone property. Do\\nNOT drive around barricades or through water of unknown depth.\\n\\nRemain out of the water due to dangerous surf conditions, or stay\\nnear occupied lifeguard towers. Rock jetties can be deadly in\\nsuch conditions, stay off the rocks.\",\n                \"response\": \"Avoid\",\n                \"parameters\": {\n                    \"AWIPSidentifier\": [\n                        \"CFWLOX\"\n                    ],\n                    \"WMOidentifier\": [\n                        \"WHUS46 KLOX 031000\"\n                    ],\n                    \"NWSheadline\": [\n                        \"HIGH SURF ADVISORY REMAINS IN EFFECT UNTIL NOON PST THURSDAY... ...COASTAL FLOOD ADVISORY REMAINS IN EFFECT UNTIL 10 AM PST THIS MORNING\"\n                    ],\n                    \"BLOCKCHANNEL\": [\n                        \"EAS\",\n                        \"NWEM\",\n                        \"CMAS\"\n                    ],\n                    \"VTEC\": [\n                        \"/O.CON.KLOX.SU.Y.0028.000000T0000Z-251204T2000Z/\"\n                    ],\n                    \"eventEndingTime\": [\n                        \"2025-12-04T12:00:00-08:00\"\n                    ],\n                    \"expiredReferences\": [\n                        \"w-nws.webmaster@noaa.gov,urn:oid:2.49.0.1.840.0.2ef03bba301f3aa5d410947a3c0b158da4ab8a14.001.1,2025-12-02T01:44:00-08:00 w-nws.webmaster@noaa.gov,urn:oid:2.49.0.1.840.0.ca1df4acb1d2f6b371b32e7cbfbf7966eb5b8a28.001.1,2025-12-01T19:11:00-08:00 w-nws.webmaster@noaa.gov,urn:oid:2.49.0.1.840.0.9f5f82a93112b0fbb919461d7f3c09a028cde467.001.2,2025-12-01T12:55:00-08:00\"\n                    ]\n                },\n                \"scope\": \"Public\",\n                \"code\": \"IPAWSv1.0\",\n                \"language\": \"en-US\",\n                \"web\": \"http://www.weather.gov\",\n                \"eventCode\": {\n                    \"SAME\": [\n                        \"NWS\"\n                    ],\n                    \"NationalWeatherService\": [\n                        \"SUY\"\n                    ]\n                }\n            }\n        },\n        {\n            \"id\": \"https://api.weather.gov/alerts/urn:oid:2.49.0.1.840.0.ecc18ad1715ddd59d073d3396e68cd94d8156f26.001.1\",\n            \"type\": \"Feature\",\n            \"geometry\": null,\n            \"properties\": {\n                \"@id\": \"https://api.weather.gov/alerts/urn:oid:2.49.0.1.840.0.ecc18ad1715ddd59d073d3396e68cd94d8156f26.001.1\",\n                \"@type\": \"wx:Alert\",\n                \"id\": \"urn:oid:2.49.0.1.840.0.ecc18ad1715ddd59d073d3396e68cd94d8156f26.001.1\",\n                \"areaDesc\": \"San Juan River Basin\",\n                \"geocode\": {\n                    \"SAME\": [\n                        \"008007\"\n                    ],\n                    \"UGC\": [\n                        \"COZ023\"\n                    ]\n                },\n                \"affectedZones\": [\n                    \"https://api.weather.gov/zones/forecast/COZ023\"\n                ],\n                \"references\": [],\n                \"sent\": \"2025-12-03T02:08:00-07:00\",\n                \"effective\": \"2025-12-03T02:08:00-07:00\",\n                \"onset\": \"2025-12-03T05:00:00-07:00\",\n                \"expires\": \"2025-12-03T17:00:00-07:00\",\n                \"ends\": \"2025-12-04T05:00:00-07:00\",\n                \"status\": \"Actual\",\n                \"messageType\": \"Alert\",\n                \"category\": \"Met\",\n                \"severity\": \"Moderate\",\n                \"certainty\": \"Likely\",\n                \"urgency\": \"Expected\",\n                \"event\": \"Winter Weather Advisory\",\n                \"sender\": \"w-nws.webmaster@noaa.gov\",\n                \"senderName\": \"NWS Grand Junction CO\",\n                \"headline\": \"Winter Weather Advisory issued December 3 at 2:08AM MST until December 4 at 5:00AM MST by NWS Grand Junction CO\",\n                \"description\": \"* WHAT...Snow expected. Total snow accumulations up to 5 inches.\\n\\n* WHERE...San Juan River Basin.\\n\\n* WHEN...Until 5 AM MST Thursday.\\n\\n* IMPACTS...Plan on slippery road conditions. The hazardous\\nconditions could impact the Wednesday morning and evening commutes.\",\n                \"instruction\": \"Slow down and use caution while traveling. The latest road\\nconditions for the state you are calling from can be obtained by\\ncalling 5 1 1.\",\n                \"response\": \"Execute\",\n                \"parameters\": {\n                    \"AWIPSidentifier\": [\n                        \"WSWGJT\"\n                    ],\n                    \"WMOidentifier\": [\n                        \"WWUS45 KGJT 030908\"\n                    ],\n                    \"NWSheadline\": [\n                        \"WINTER WEATHER ADVISORY IN EFFECT UNTIL 5 AM MST THURSDAY\"\n                    ],\n                    \"BLOCKCHANNEL\": [\n                        \"EAS\",\n                        \"NWEM\",\n                        \"CMAS\"\n                    ],\n                    \"VTEC\": [\n                        \"/O.EXB.KGJT.WW.Y.0026.251203T1200Z-251204T1200Z/\"\n                    ],\n                    \"eventEndingTime\": [\n                        \"2025-12-04T05:00:00-07:00\"\n                    ]\n                },\n                \"scope\": \"Public\",\n                \"code\": \"IPAWSv1.0\",\n                \"language\": \"en-US\",\n                \"web\": \"http://www.weather.gov\",\n                \"eventCode\": {\n                    \"SAME\": [\n                        \"NWS\"\n                    ],\n                    \"NationalWeatherService\": [\n                        \"WWY\"\n                    ]\n                }\n            }\n        },\n        {\n            \"id\": \"https://api.weather.gov/alerts/urn:oid:2.49.0.1.840.0.ecc18ad1715ddd59d073d3396e68cd94d8156f26.003.1\",\n            \"type\": \"Feature\",\n            \"geometry\": null,\n            \"properties\": {\n                \"@id\": \"https://api.weather.gov/alerts/urn:oid:2.49.0.1.840.0.ecc18ad1715ddd59d073d3396e68cd94d8156f26.003.1\",\n                \"@type\": \"wx:Alert\",\n                \"id\": \"urn:oid:2.49.0.1.840.0.ecc18ad1715ddd59d073d3396e68cd94d8156f26.003.1\",\n                \"areaDesc\": \"Grand and Battlement Mesas; West Elk and Sawatch Mountains; Uncompahgre Plateau/Dallas Divide\",\n                \"geocode\": {\n                    \"SAME\": [\n                        \"008029\",\n                        \"008045\",\n                        \"008077\",\n                        \"008051\",\n                        \"008085\",\n                        \"008091\",\n                        \"008113\"\n                    ],\n                    \"UGC\": [\n                        \"COZ009\",\n                        \"COZ012\",\n                        \"COZ017\"\n                    ]\n                },\n                \"affectedZones\": [\n                    \"https://api.weather.gov/zones/forecast/COZ009\",\n                    \"https://api.weather.gov/zones/forecast/COZ012\",\n                    \"https://api.weather.gov/zones/forecast/COZ017\"\n                ],\n                \"references\": [\n                    {\n                        \"@id\": \"https://api.weather.gov/alerts/urn:oid:2.49.0.1.840.0.1e2e3f318117076bbf552163bdfe24a72a2e2d99.001.1\",\n                        \"identifier\": \"urn:oid:2.49.0.1.840.0.1e2e3f318117076bbf552163bdfe24a72a2e2d99.001.1\",\n                        \"sender\": \"w-nws.webmaster@noaa.gov\",\n                        \"sent\": \"2025-12-02T17:12:00-07:00\"\n                    }\n                ],\n                \"sent\": \"2025-12-03T02:08:00-07:00\",\n                \"effective\": \"2025-12-03T02:08:00-07:00\",\n                \"onset\": \"2025-12-03T02:08:00-07:00\",\n                \"expires\": \"2025-12-03T17:00:00-07:00\",\n                \"ends\": \"2025-12-04T02:00:00-07:00\",\n                \"status\": \"Actual\",\n                \"messageType\": \"Update\",\n                \"category\": \"Met\",\n                \"severity\": \"Moderate\",\n                \"certainty\": \"Likely\",\n                \"urgency\": \"Expected\",\n                \"event\": \"Winter Weather Advisory\",\n                \"sender\": \"w-nws.webmaster@noaa.gov\",\n                \"senderName\": \"NWS Grand Junction CO\",\n                \"headline\": \"Winter Weather Advisory issued December 3 at 2:08AM MST until December 4 at 2:00AM MST by NWS Grand Junction CO\",\n                \"description\": \"* WHAT...Snow. Additional snow accumulations between 3 and 6 inches.\\n\\n* WHERE...Grand and Battlement Mesas, Uncompahgre Plateau and Dallas\\nDivide, and West Elk and Sawatch Mountains.\\n\\n* WHEN...Until 2 AM MST Thursday.\\n\\n* IMPACTS...Travel could be very difficult. The hazardous conditions\\ncould impact the Wednesday morning and evening commutes.\",\n                \"instruction\": \"Slow down and use caution while traveling. The latest road\\nconditions for the state you are calling from can be obtained by\\ncalling 5 1 1.\",\n                \"response\": \"Execute\",\n                \"parameters\": {\n                    \"AWIPSidentifier\": [\n                        \"WSWGJT\"\n                    ],\n                    \"WMOidentifier\": [\n                        \"WWUS45 KGJT 030908\"\n                    ],\n                    \"NWSheadline\": [\n                        \"WINTER WEATHER ADVISORY REMAINS IN EFFECT UNTIL 2 AM MST THURSDAY\"\n                    ],\n                    \"BLOCKCHANNEL\": [\n                        \"EAS\",\n                        \"NWEM\",\n                        \"CMAS\"\n                    ],\n                    \"VTEC\": [\n                        \"/O.CON.KGJT.WW.Y.0026.000000T0000Z-251204T0900Z/\"\n                    ],\n                    \"eventEndingTime\": [\n                        \"2025-12-04T02:00:00-07:00\"\n                    ]\n                },\n                \"scope\": \"Public\",\n                \"code\": \"IPAWSv1.0\",\n                \"language\": \"en-US\",\n                \"web\": \"http://www.weather.gov\",\n                \"eventCode\": {\n                    \"SAME\": [\n                        \"NWS\"\n                    ],\n                    \"NationalWeatherService\": [\n                        \"WWY\"\n                    ]\n                }\n            }\n        },\n        {\n            \"id\": \"https://api.weather.gov/alerts/urn:oid:2.49.0.1.840.0.ecc18ad1715ddd59d073d3396e68cd94d8156f26.005.1\",\n            \"type\": \"Feature\",\n            \"geometry\": null,\n            \"properties\": {\n                \"@id\": \"https://api.weather.gov/alerts/urn:oid:2.49.0.1.840.0.ecc18ad1715ddd59d073d3396e68cd94d8156f26.005.1\",\n                \"@type\": \"wx:Alert\",\n                \"id\": \"urn:oid:2.49.0.1.840.0.ecc18ad1715ddd59d073d3396e68cd94d8156f26.005.1\",\n                \"areaDesc\": \"Southwest San Juan Mountains\",\n                \"geocode\": {\n                    \"SAME\": [\n                        \"008007\",\n                        \"008033\",\n                        \"008053\",\n                        \"008067\",\n                        \"008083\",\n                        \"008111\",\n                        \"008113\"\n                    ],\n                    \"UGC\": [\n                        \"COZ019\"\n                    ]\n                },\n                \"affectedZones\": [\n                    \"https://api.weather.gov/zones/forecast/COZ019\"\n                ],\n                \"references\": [\n                    {\n                        \"@id\": \"https://api.weather.gov/alerts/urn:oid:2.49.0.1.840.0.59f7bbb1b05f341c96e55d508e395b781ba80eb6.001.1\",\n                        \"identifier\": \"urn:oid:2.49.0.1.840.0.59f7bbb1b05f341c96e55d508e395b781ba80eb6.001.1\",\n                        \"sender\": \"w-nws.webmaster@noaa.gov\",\n                        \"sent\": \"2025-12-02T12:59:00-07:00\"\n                    },\n                    {\n                        \"@id\": \"https://api.weather.gov/alerts/urn:oid:2.49.0.1.840.0.1e2e3f318117076bbf552163bdfe24a72a2e2d99.004.1\",\n                        \"identifier\": \"urn:oid:2.49.0.1.840.0.1e2e3f318117076bbf552163bdfe24a72a2e2d99.004.1\",\n                        \"sender\": \"w-nws.webmaster@noaa.gov\",\n                        \"sent\": 
